vi "Scale_To_Range(2D).vi"(9 "min pixel score":sgl, 10 "max pixel score":sgl, 11 "anomaly map":sgl[][](array[numeric])) -> (3 "anomaly map normalized":sgl[][](array[numeric]))   [LabVIEW 2024]
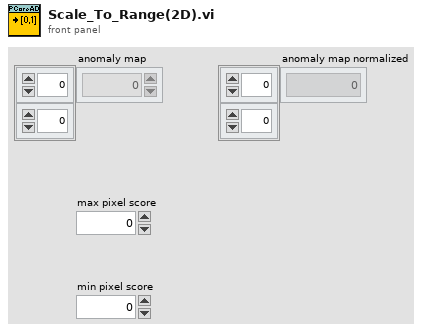
[diagram p1: front panel]
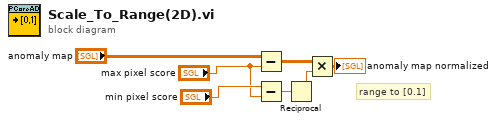
[diagram p0: block diagram]
diagram:
  # "range to [0.1]"
  n1 = Subtract(x="anomaly map", y="max pixel score") -> (x-y=w3:sgl[][])
  n2 = Subtract(x="min pixel score", y="max pixel score") -> (x-y=w4:sgl)
  n3 = Reciprocal(x=w4) -> (1/x=w1:sgl)
  n4 = Multiply(x=w3, y=w1) -> (x*y=→"anomaly map normalized":sgl[][])
